vi "WriteFile.vi"(9 "Write?":bool=TRUE, 10 "Data":string[](array[string]), 11 "Path":path) -> ()   [LabVIEW 2024]
uses:
  <vilib>/Utility/file.llb/Write Delimited Spreadsheet (string).vi
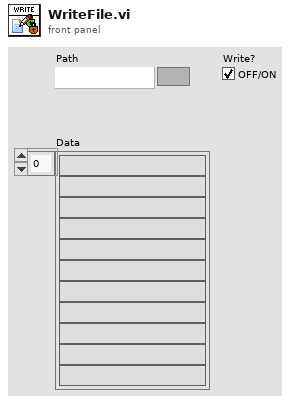
[diagram p1: front panel]
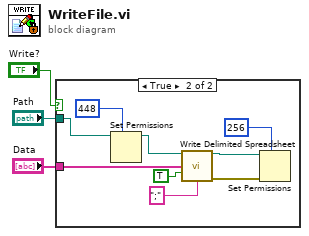
[diagram p0: block diagram]
diagram:
  n1 = case shown="True" "Write?" {
    tunnel: "Path" -> [_ w9]
    tunnel: "Data" -> [_ w10]
    frame False {
    }
    frame True {
      n2 = Set Permissions(7:i16 448 ("permissions"), 11:w9) -> (3:w8:path)  [unwired: 3 in, 1 out]
      n3 = call-poly <vilib>:"Write Delimited Spreadsheet.vi"("file path (dialog if empty)"=w8, "1D data"=w10, "append to file? (new file:F)"=TRUE, "delimiter (\\t)"=";" ("delimiter (\\t)")) -> ("new file path (Not A Path if cancelled)"=w7:path, "error out"=w6:errorcluster)  [unwired: 10 in]
      n4 = Set Permissions(7:i16 256 ("permissions"), 8:w6, 11:w7) -> ()  [unwired: 2 in, 2 out]
    }
  }
